vi "BusOut_read.vi"(8 "error in (no error)":errorcluster, 11 "BusOut in":refnum<class "BusOut.lvclass">) -> (0 "error out":errorcluster, 2 "value":dbl, 3 "BusOut out":refnum<class "BusOut.lvclass">)   [LabVIEW 2011, in "mbed_LVLibrary.lvlib" / "BusOut.lvclass"]
uses:
  BusOut.lvclass
  BusOut.lvclass/BusOut.ctl
  Transport Mechanisms/mbed/mbed.lvclass
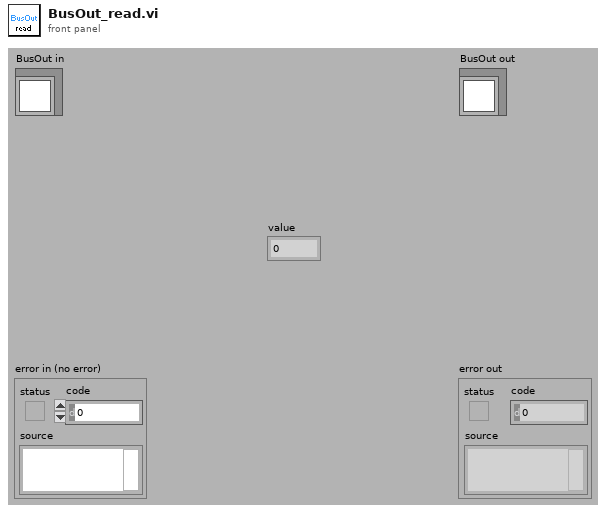
[diagram p1: front panel]
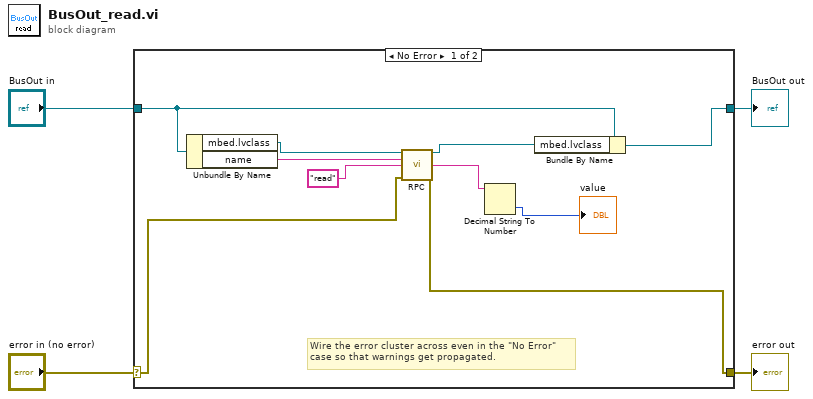
[diagram p0: block diagram]
diagram:
  n1 = case shown="No Error" "error in (no error)" {
    selector: "error in (no error)" -> [w6 w16]
    tunnel: [w5 w16] -> w3
    tunnel: [w13 w15] -> w1
    tunnel: "BusOut in" -> [w14 w15]
    frame No Error {
      # "Wire the error cluster across even in the \"No Error\"\ncase so that warnings get propagated."
      n2 = Unbundle By Name(w14) -> ("mbed.lvclass"=w12:refnum<class "mbed.lvclass">, "name"=w11:string)
      n3 = call-dynamic "RPC.vi"("mbed in"=w12, "Name"=w11, "method"="read", "error in (no error)"=w6) -> ("mbed out"=w10:refnum<class "mbed.lvclass">, "RPC Result"=w7:string, "error out"=w5:errorcluster)  [unwired: 9 in]
      n4 = Decimal String To Number(string=w7) -> (number=→"value":i32)  [unwired: 2 in, 1 out]
      n5 = Bundle By Name(cluster=w14, "mbed.lvclass"=w10) -> (w13:refnum<class "BusOut.lvclass">)
    }
    frame Error {
    }
  }
  "error out" <- w3
  "BusOut out" <- w1
